vi "Telemetry Receiver.vi"   [LabVIEW 2020]
types:
  T1 = typedef "Data Frame.ctl" = cluster{"Frame Header":T2, "Payload":string, "CRC":u32}
  T2 = typedef "Data Frame Header.ctl" = cluster{"Sync":u32, "Time":dbl, "Nanosecond Counter":i64, "Payload Class":T3, "Payload ID":u16, "Counter":u32, "Options":u32, "Source":i32, "Destination":i32}
  T3 = typedef "Payload Class.ctl" = enum16{"System State", "Parameters", "Metadata", "Software Monitor", "Data", "Commands"}
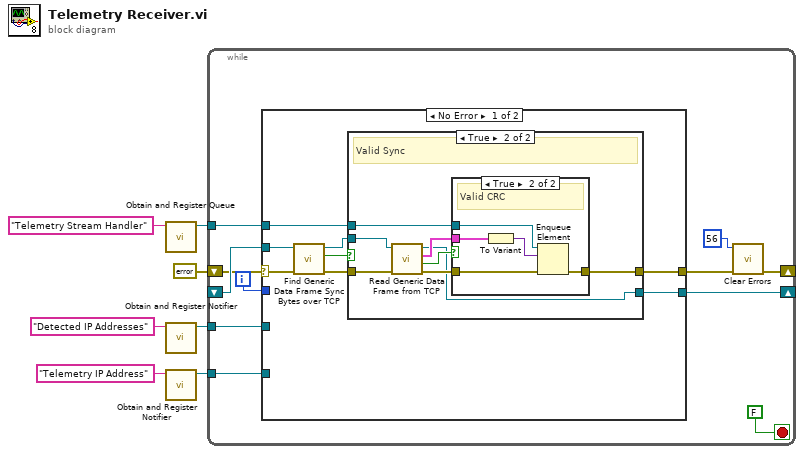
[diagram p0: block diagram]
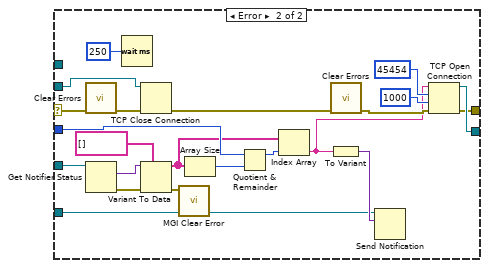
[diagram p4: hidden frame]
diagram:
  n1 = call "Obtain and Register Queue.vi"("name (unnamed)"="Telemetry Stream Handler") -> ("Queue Out"=w3:refnum<queue>)  [unwired: 7 in, 3 out]
  n2 = call "Obtain and Register Notifier.vi"("name (unnamed)"="Detected IP Addresses") -> ("notifier out"=w5:refnum<notifier>)  [unwired: 8 in, 2 out]
  n3 = call "Obtain and Register Notifier.vi"("name (unnamed)"="Telemetry IP Address") -> ("notifier out"=w7:refnum<notifier>)  [unwired: 8 in, 2 out]
  n4 = while {
    shift-right: [w8] -> _
    shift-left: errorcluster {"status"=TRUE, "code"=0, "source"=""} ("error in (no error)") -> [w14]
    shift-right: [w18] -> _
    shift-left: _ -> [w17]
    tunnel: w3 -> [w15]
    tunnel: w5 -> [w12]
    tunnel: w7 -> [w11]
    i -> [w13]
    stop <- FALSE stop-if-true
    n5 = case shown="No Error" w14 {
      selector: w14 -> [w26 w64]
      tunnel: [w21 w57] -> w9
      tunnel: [w23 w59] -> w18
      tunnel: w17 -> [w25 w60]
      tunnel: w15 -> [w19 _]
      tunnel: w13 -> [_ w52]
      tunnel: w12 -> [_ w49]
      tunnel: w11 -> [_ w44]
      frame No Error {
        n6 = call "Find Generic Data Frame Sync Bytes over TCP.vi"("error in (no error)"=w26, "TCP Network Connection in"=w25) -> ("error out"=w22:errorcluster, "Valid Sync"=w20:bool, "TCP Network Connection out"=w24:refnum<k5>)  [unwired: 7 in]
        n7 = case shown="True" w20 {
          tunnel: w24 -> [w28 w36]
          tunnel: [w28 w29] -> w23
          tunnel: w22 -> [w27 w35]
          tunnel: [w27 w30] -> w21
          tunnel: w19 -> [_ w32]
          frame False {
            # "Invalid Sync"
          }
          frame True {
            # "Valid Sync"
            n8 = call "Read Generic Data Frame from TCP.vi"("error in (no error)"=w35, "TCP Network Connection in"=w36) -> ("error out"=w31:errorcluster, "Valid CRC"=w33:bool, "Frame Received"=w34:T1, "TCP Network Connection out"=w29:refnum<k5>)  [unwired: 6 in]
            n9 = case shown="True" w33 {
              tunnel: w34 -> [_ w38]
              tunnel: w32 -> [_ w42]
              tunnel: w31 -> [w37 w41]
              tunnel: [w37 w40] -> w30
              frame False {
                # "Invalid CRC"
              }
              frame True {
                # "Valid CRC"
                n10 = To Variant(anything=w38) -> (Variant=w39:variant)
                n11 = Enqueue Element(queue=w42, element=w39, error in (no error)=w41) -> (error out=w40:errorcluster)  [unwired: 1 in, 2 out]
              }
            }
          }
        }
      }
      frame Error {
        n12 = call <vilib>:"Clear Errors.vi"("error in (no error)"=w64) -> ("error out"=w62:errorcluster)  [unwired: 5 in, 1 out]
        n13 = Get Notifier Status(notifier=w49) -> (current notification=w51:variant, error out=w47:errorcluster)  [unwired: 1 in, 3 out]
        n14 = Wait (ms)(milliseconds to wait=u32 250) -> ()  [unwired: 1 out]
        n15 = TCP Close Connection(connection ID=w60, error in (no error)=w62) -> (error out=w61:errorcluster)  [unwired: 1 in, 1 out]
        n16 = Variant To Data(error in=w47, type=string[] [] ("Adapter IP Addresses"), Variant=w51) -> (data=w48:string[], error out=w46:errorcluster)
        n17 = call <userlib>:"MGI Clear Error.vi"("Error In"=w46) -> ()  [unwired: 6 in, 1 out]
        n18 = Array Size(array=w48) -> (size(s)=w53:i32)
        n19 = Quotient & Remainder(x=w52, y=w53) -> (x-y*floor(x/y)=w54:i32)  [unwired: 1 out]
        n20 = Index Array(array=w48, index=w54) -> (element=w43:string)
        n21 = call <vilib>:"Clear Errors.vi"("error in (no error)"=w61) -> ("error out"=w58:errorcluster)  [unwired: 5 in, 1 out]
        n22 = To Variant(anything=w43) -> (Variant=w45:variant)
        n23 = Send Notification(notification=w45, notifier=w44) -> ()  [unwired: 1 in, 2 out]
        n24 = TCP Open Connection(address=w43, remote port or service name=u16 45454 ("port"), timeout ms (60000)=1000 ("timeout ms (wait forever: -1)"), error in (no error)=w58) -> (connection ID=w59:refnum<k5>, error out=w57:errorcluster)  [unwired: 1 in]
      }
    }
    n25 = call <vilib>:"Clear Errors.vi"("error in (no error)"=w9, "specific error code to clear (0: all)"=56) -> ("error out"=w8:errorcluster)  [unwired: 4 in, 1 out]
  }
